vi "Measure uWave Range.vi"(8 "error in (no error)":errorcluster, 11 "MWWL Verification in":refnum<class "MWWL Verification.lvclass">) -> (0 "error out":errorcluster, 3 "MWWL Verification out":refnum<class "MWWL Verification.lvclass">)   [LabVIEW 2018, in "MWWL Verification.lvlib" / "MWWL Verification.lvclass"]
uses:
  MWWL Verification.lvclass
  MWWL Verification.lvclass/MWWL Verification.ctl
  <vilib>/ActorFramework/Message Enqueuer/Message Enqueuer.lvclass/Message Enqueuer.ctl
  <vilib>/ActorFramework/Message Enqueuer/Enqueue.vi
  H3611i Actor/H3611i Actor Messages/Measure H3611i Range Msg/Measure H3611i Range Msg.lvclass
  C:/Program Files (x86)/National Instruments/LabVIEW 2018/vi.lib/ActorFramework/Message/Message.lvclass
  <vilib>/ActorFramework/Message Priority Queue/Priority Enqueue.vi
panel:
  in  "H3611i?":bool
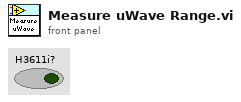
[diagram p1: front panel]
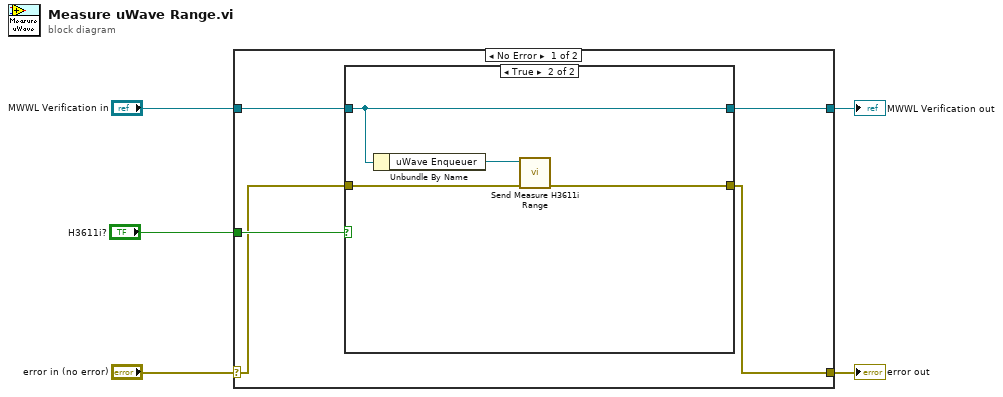
[diagram p0: block diagram]
diagram:
  n1 = case shown="No Error" "error in (no error)" {
    selector: "error in (no error)" -> [w7 w18]
    tunnel: [w6 w18] -> w4
    tunnel: [w8 w17] -> w2
    tunnel: "MWWL Verification in" -> [w9 w17]
    tunnel: "H3611i?" -> [w10 _]
    frame No Error {
      n2 = case shown="True" w10 {
        tunnel: w9 -> [w12 w16]
        tunnel: [w12 w16] -> w8
        tunnel: w7 -> [w11 w14]
        tunnel: [w11 w13] -> w6
        frame False {
        }
        frame True {
          n3 = Unbundle By Name(w16) -> ("uWave Enqueuer"=w15:refnum<class "Message Enqueuer.lvclass">)
          n4 = call "Send Measure H3611i Range.vi"("error in (no error)"=w14, "Message Enqueuer in"=w15) -> ("error out"=w13:errorcluster)  [unwired: 8 in, 1 out]
        }
      }
    }
    frame Error {
    }
  }
  "error out" <- w4
  "MWWL Verification out" <- w2
